vi "Read Analog Input.vi"(8 "error in (no error)":errorcluster, 10 "Node (3)":u8=3 caption="Node" min=3 max=128 step=1, 11 "VISA resource name":refnum<visa-resource-name>) -> (0 "error out":errorcluster, 2 "Analog Input Value":i16 caption="Analog Input", 3 "VISA resource name out":refnum<visa-resource-name>)   [LabVIEW 2019, in "Bronkhorst FLOW-BUS.lvlib"]
doc: "Reads the analog input on the device. Depending on the analog mode, the signal (0...5Vdc / 0…10Vdc / 0...20mA / 4...20mA) is converted to a value between 0 and 32000.\nAnalog input signals (digitized) are in the same range as measured values (0...32000 = 0...100%)."
uses:
  Bronkhorst FLOW-BUS.lvlib
  Private/FLOW-BUS RW.ctl
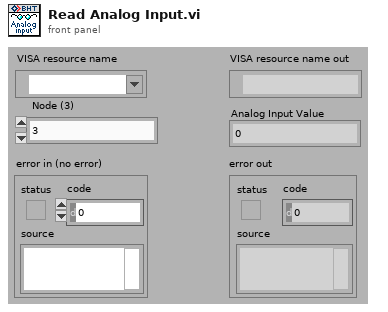
[diagram p1: front panel]
types:
  T1 = typedef "Bronkhorst FLOW-BUS.lvlib/FLOW-BUS RW.ctl" = cluster{"Node Address (3)":u8, "Communication Command":enum16{"Status message", "Send parameter with destination address and 00 response", "Send parameter with destination address", "Request parameter"}, "Process (0)":u16, "Parameter (0)":u16, "Data Type (0: Character)":enum16{"Character", "Integer", "Float or Long", "String"}, "Data for Char or Int (0)":u32, "Data for Float or Long (0)":sgl, "Data for String":string, "Length of Requested String (0)":u8}
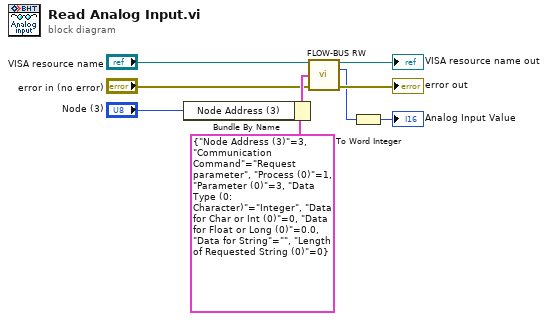
[diagram p0: block diagram]
diagram:
  n1 = Bundle By Name(cluster=T1 {"Node Address (3)"=3, "Communication Command"=enum."Request parameter", "Process (0)"=1, "Parameter (0)"=3, "Data Type (0: Character)"=enum."Integer", "Data for Char or Int (0)"=0, "Data for Float or Long (0)"=0.0, "Data for String"="", "Length of Requested String (0)"=0} ("FLOW-BUS Command Settings"), "Node Address (3)"="Node (3)") -> (w9:T1)
  n2 = call "FLOW-BUS RW.vi"("VISA resource name"="VISA resource name", "FLOW-BUS Command Settings"=w9, "error in (no error)"="error in (no error)") -> ("VISA resource name out"=→"VISA resource name out":refnum<visa-resource-name>, "Requested Char, Int or Long"=w2:u32, "error out"=→"error out":errorcluster)  [unwired: 8 in, 2 out]
  n3 = To Word Integer(number=w2) -> (16bit integer=→"Analog Input Value":i16)
